vi "IsUserInputInRange.vi"(11 "User Input in":T1) -> (3 "InRange?":bool)   [LabVIEW 2017]
uses:
  Ctrl/UserInput.ctl
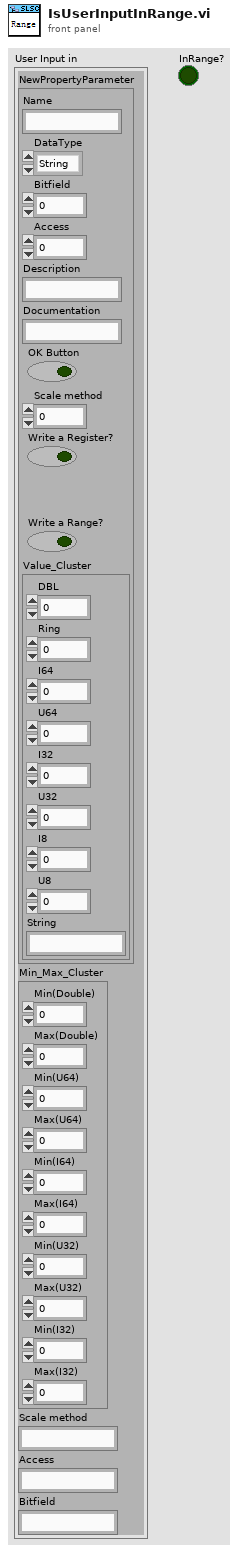
[diagram p1: front panel]
types:
  T1 = typedef "UserInput.ctl" = cluster{"NewPropertyParameter":cluster{"Name":string, "DataType":enum16{"String", "Double", "U64", "I64", "U32", "I32", "Bool"}, "Bitfield":u16, "Access":u16, "Description":string, "Documentation":string, "OK Button":bool, "Scale method":u16, "Write a Register?":bool, "Write a Range?":bool, "Value_Cluster":cluster{"DBL":dbl, "Ring":u16, "I64":i64, "U64":u64, "I32":i32, "U32":u32, "I8":i8, "U8":u8, "String":string}}, "Min_Max_Cluster":cluster{"Min(Double)":dbl, "Max(Double)":dbl, "Min(U64)":u64, "Max(U64)":u64, "Min(I64)":i64, "Max(I64)":i64, "Min(U32)":u32, "Max(U32)":u32, "Min(I32)":i32, "Max(I32)":i32}, "Scale method":string, "Access":string, "Bitfield":string}
  T2 = cluster{"DBL":dbl, "Ring":u16, "I64":i64, "U64":u64, "I32":i32, "U32":u32, "I8":i8, "U8":u8, "String":string}
  T3 = enum16{"String", "Double", "U64", "I64", "U32", "I32", "Bool"}
  T4 = cluster{"Min(Double)":dbl, "Max(Double)":dbl, "Min(U64)":u64, "Max(U64)":u64, "Min(I64)":i64, "Max(I64)":i64, "Min(U32)":u32, "Max(U32)":u32, "Min(I32)":i32, "Max(I32)":i32}
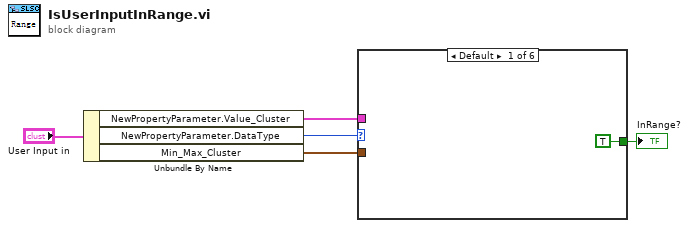
[diagram p0: block diagram]
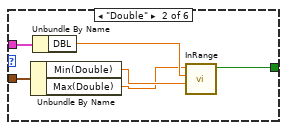
[diagram p2: hidden frame]
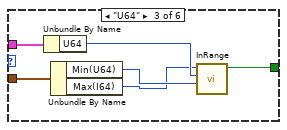
[diagram p3: hidden frame]
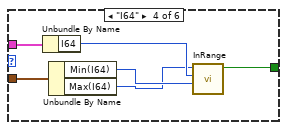
[diagram p4: hidden frame]
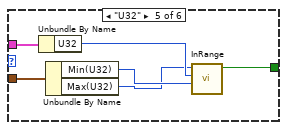
[diagram p5: hidden frame]
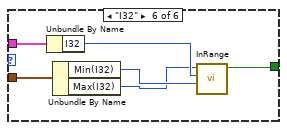
[diagram p6: hidden frame]
diagram:
  n1 = Unbundle By Name("User Input in") -> ("NewPropertyParameter.Value_Cluster"=w4:T2, "NewPropertyParameter.DataType"=w2:T3, "Min_Max_Cluster"=w3:T4)
  n2 = case shown="Default" w2 {
    tunnel: w3 -> [_ w11 w14 w20 w26 w32]
    tunnel: w4 -> [_ w12 w15 w21 w27 w33]
    tunnel: [TRUE ("Boolean") w7 w13 w19 w25 w31] -> w5
    frame Default {
    }
    frame "Double" {
      n3 = Unbundle By Name(w11) -> ("Min(Double)"=w9:dbl, "Max(Double)"=w8:dbl)
      n4 = Unbundle By Name(w12) -> ("DBL"=w10:dbl)
      n5 = call "InRange.vi"("Min"=w9, "Value"=w10, "Max"=w8) -> ("Boolean"=w7:bool)  [unwired: 8 in]
    }
    frame "U64" {
      n6 = Unbundle By Name(w15) -> ("U64"=w18:u64)
      n7 = Unbundle By Name(w14) -> ("Min(U64)"=w17:u64, "Max(I64)"=w16:i64)
      n8 = call "InRange.vi"("Min"=w17, "Value"=w18, "Max"=w16) -> ("Boolean"=w13:bool)  [unwired: 8 in]
    }
    frame "I64" {
      n9 = Unbundle By Name(w21) -> ("I64"=w24:i64)
      n10 = Unbundle By Name(w20) -> ("Min(I64)"=w23:i64, "Max(I64)"=w22:i64)
      n11 = call "InRange.vi"("Min"=w23, "Value"=w24, "Max"=w22) -> ("Boolean"=w19:bool)  [unwired: 8 in]
    }
    frame "U32" {
      n12 = Unbundle By Name(w27) -> ("U32"=w30:u32)
      n13 = Unbundle By Name(w26) -> ("Min(U32)"=w29:u32, "Max(U32)"=w28:u32)
      n14 = call "InRange.vi"("Min"=w29, "Value"=w30, "Max"=w28) -> ("Boolean"=w25:bool)  [unwired: 8 in]
    }
    frame "I32" {
      n15 = Unbundle By Name(w33) -> ("I32"=w36:i32)
      n16 = Unbundle By Name(w32) -> ("Min(I32)"=w35:i32, "Max(I32)"=w34:i32)
      n17 = call "InRange.vi"("Min"=w35, "Value"=w36, "Max"=w34) -> ("Boolean"=w31:bool)  [unwired: 8 in]
    }
  }
  "InRange?" <- w5
